vi "Keithley 6514 Read Limits Results.vi"(0 "Resource In":refnum<visa-resource-name>, 1 "Check For SCPI Errors? (T)":bool=TRUE, 11 "error in":T1) -> (4 "Resource Out (dupl)":refnum<visa-resource-name>, 6 "Limits 1 Pass?":bool, 8 "Limits 2 Pass?":bool, 15 "error out":T1)   [LabVIEW 2014, in "KE6514Driver.lvlib"]
doc: "This VI is used to read the results of the Limits Test."
uses:
  KE6514Driver.lvlib
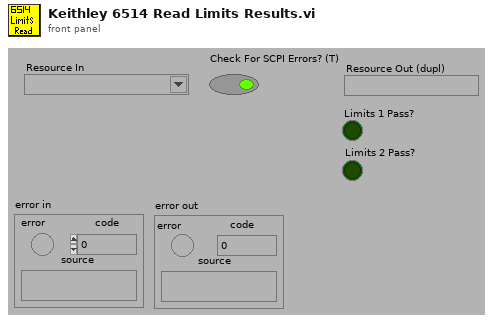
[diagram p1: front panel]
types:
  T1 = cluster{"error":bool, "code":i32, "source":string}
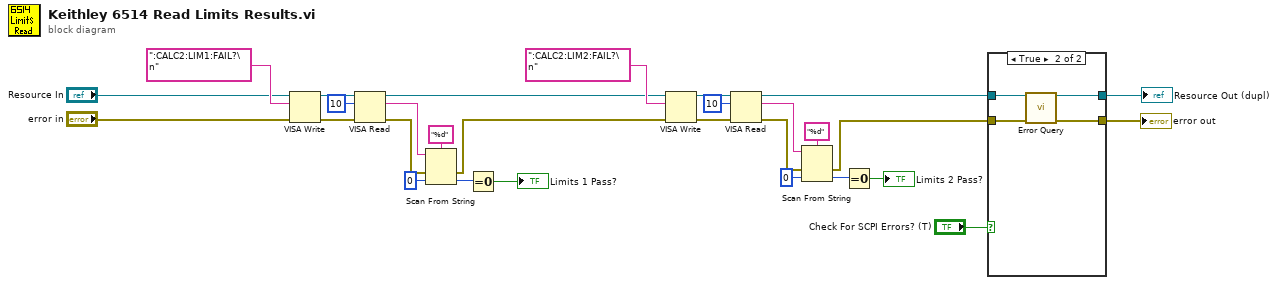
[diagram p0: block diagram]
diagram:
  n1 = VISA Write(VISA resource name="Resource In", write buffer=":CALC2:LIM1:FAIL?\n", error in (no error)="error in") -> (VISA resource name out=w26:refnum<visa-resource-name>, error out=w24:errorcluster)  [unwired: 1 out]
  n2 = VISA Read(VISA resource name=w26, byte count=u32 10, error in (no error)=w24) -> (VISA resource name out=w8:refnum<visa-resource-name>, read buffer=w20:string, error out=w21:errorcluster)  [unwired: 1 out]
  n3 = Scan From String(format string="%d", input string=w20, error in=w21, default 1=0 ("default value 1")) -> (error out=w7:errorcluster, output 1=w22:i32)  [unwired: 1 in, 2 out]
  n4 = Equal To 0?(x=w22) -> (x = 0?=→"Limits 1 Pass?":bool)
  n5 = VISA Write(VISA resource name=w8, write buffer=":CALC2:LIM2:FAIL?\n", error in (no error)=w7) -> (VISA resource name out=w16:refnum<visa-resource-name>, error out=w14:errorcluster)  [unwired: 1 out]
  n6 = VISA Read(VISA resource name=w16, byte count=u32 10, error in (no error)=w14) -> (VISA resource name out=w4:refnum<visa-resource-name>, read buffer=w10:string, error out=w11:errorcluster)  [unwired: 1 out]
  n7 = Scan From String(format string="%d", input string=w10, error in=w11, default 1=0 ("default value 1")) -> (error out=w3:errorcluster, output 1=w12:i32)  [unwired: 1 in, 2 out]
  n8 = Equal To 0?(x=w12) -> (x = 0?=→"Limits 2 Pass?":bool)
  n9 = case shown="True" "Check For SCPI Errors? (T)" {
    tunnel: w4 -> [w31 w35]
    tunnel: w3 -> [w30 w34]
    tunnel: [w30 w33] -> w1
    tunnel: [w31 w32] -> w2
    frame False {
    }
    frame True {
      n10 = call "Error Query.vi"("VISA Resource In"=w35, "error in (no error)"=w34) -> ("VISA Resource Out (dupl)"=w32:refnum<visa-resource-name>, "error out"=w33:errorcluster)  [unwired: 10 in, 2 out]
    }
  }
  "error out" <- w1
  "Resource Out (dupl)" <- w2
